vi "sendTwitterCellStats.vi"(8 "error in":errorcluster, 9 "Prev Phase":string, 10 "Prev Exp":T1(ring)=enum."Current Pulse", 11 "cell stats":T2 {"STD" format="%010.2f"; "Variance" format="%010.2f"; "Rt (MOhms)" format="%010.2f"; "tau (ms)" format="%08.2g"; "Cm (pF)" format="%08.2f"; "Ra (MOhms)" format="%010.2f"; "Rm (MOhms)" format="%010.2f"; "Ihold (pA)" format="%010.2f"}) -> (0 "error out":errorcluster, 3 "check Time":timestamp)   [LabVIEW 2019]
uses:
  <vilib>/LVH/i3 Twitter/Controls/Twitter Handle.ctl
  <vilib>/LVH/i3 OAuth/Controls/OAuth Handle.ctl
  <vilib>/LVH/i3 OAuth/Controls/Signature Method.ctl
  <vilib>/LVH/i3 OAuth/Controls/Credentials.ctl
  wc_protocol_v1.003 Folder/whole_cell_protocol/Controls/cell_stats-v02.ctl
  <vilib>/LVH/i3 Twitter/SubVIs/Twitter Open - Embedded.vi
  <vilib>/LVH/i3 Twitter/Tweets/Post Tweet.vi
  <vilib>/LVH/i3 Twitter/i3-twitter.lvlib
  <vilib>/LVH/i3 OAuth/i3-oauth.lvlib
panel:
  out "tweet sent":string
  out "Twitter Handle Out":T3={"OAuth Credentials"={"Signature Method"=enum."HMAC-SHA1", "Version"="1.0", "Client"={"Token"="", "Secret"=""}, "Access"={"Token"="", "Secret"=""}}, "since ID"="", "max ID"="", "Screen Name"=""}
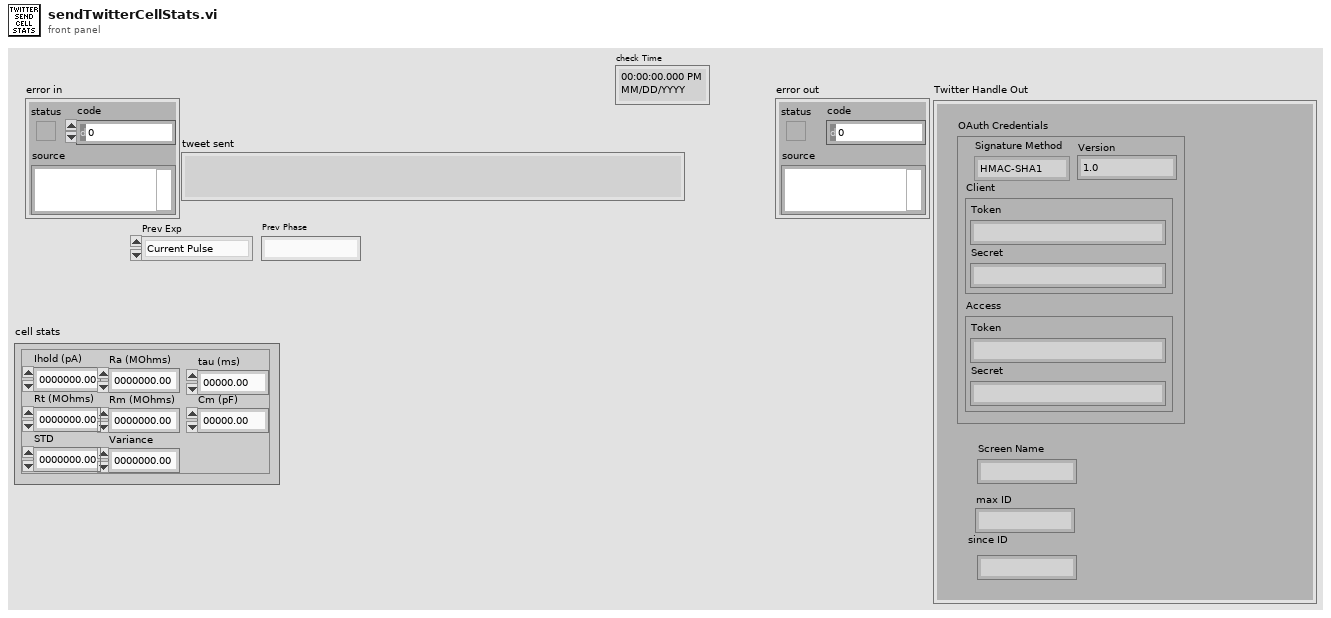
[diagram p1: front panel]
types:
  T1 = enum32{"Single Jump", "Solution Change", "Voltage Step", "Voltage Ramp", "Voltage Pulse", "Jump Train", "Paired Pulse", "Single Manip Jump", "Gap Free", "Multi M. Jump", "Current Pulse", "Current Ramp", "Gap Free Iclamp"}
  T2 = typedef "cell_stats-v02.ctl" = cluster{"Ihold (pA)":dbl, "Rm (MOhms)":dbl, "Ra (MOhms)":dbl, "Cm (pF)":dbl, "tau (ms)":dbl, "Rt (MOhms)":dbl, "Variance":dbl, "STD":dbl}
  T3 = typedef "i3-twitter.lvlib/Twitter Handle.ctl" = cluster{"OAuth Credentials":T4, "since ID":string, "max ID":string, "Screen Name":string}
  T4 = typedef "i3-oauth.lvlib/OAuth Handle.ctl" = cluster{"Signature Method":T5, "Version":string, "Client":T6, "Access":T6}
  T5 = typedef "i3-oauth.lvlib/Signature Method.ctl" = enum16{"HMAC-MD5", "HMAC-SHA1", "HMAC-SHA224", "HMAC-SHA256", "HMAC-SHA384", "HMAC-SHA512"}
  T6 = typedef "i3-oauth.lvlib/Credentials.ctl" = cluster{"Token":string, "Secret":string}
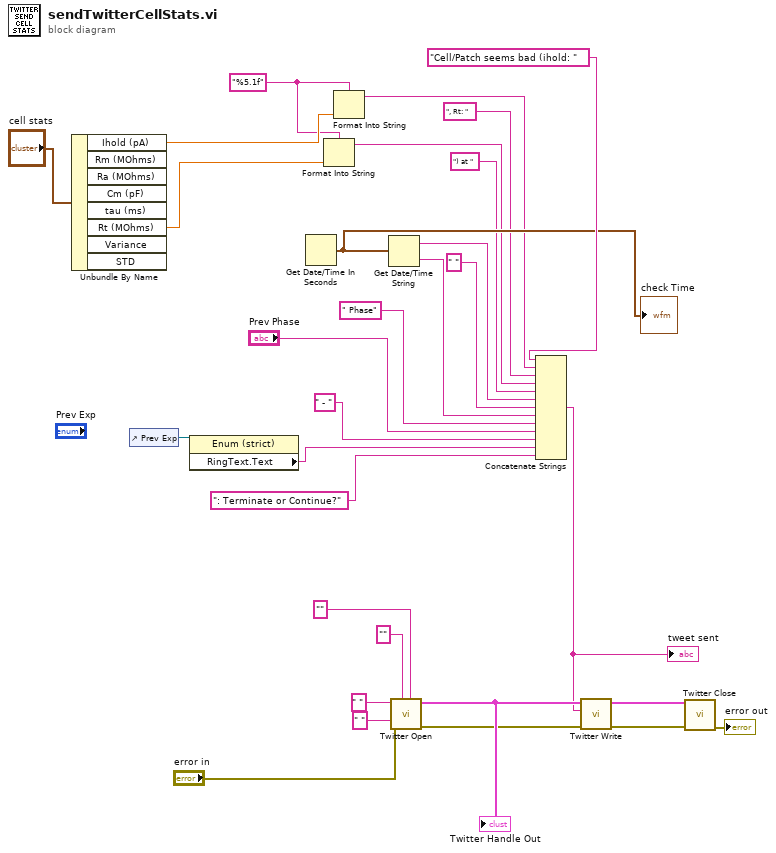
[diagram p0: block diagram]
diagram:
  w1 = "%5.1f" ("format string")
  n1 = Unbundle By Name("cell stats") -> ("Ihold (pA)"=w13:dbl, "Rt (MOhms)"=w11:dbl)  [unwired: 6 out]
  n2 = control-ref of="Prev Exp"() -> (w4:refnum<vi>)
  n3 = property class="Enum (strict)"(reference=w4) -> ("RingText.Text"=w3:string)  [unwired: 1 in, 2 out]
  n4 = Get Date/Time In Seconds() -> (seconds since 1Jan1904=w18:timestamp)
  "check Time" <- w18
  n5 = Format Into String(format string=w1, w11) -> (resulting string=w10:string)  [unwired: 2 in, 1 out]
  n6 = Format Into String(format string=w1, w13) -> (resulting string=w12:string)  [unwired: 2 in, 1 out]
  n7 = Get Date/Time String(seconds (now)=w18) -> (date string=w17:string, time string=w16:string)  [unwired: 2 in]
  n8 = call-poly <vilib>:"Twitter Open.vi"("Access Secret"="", "Access Token"="", "error in"="error in", "Consumer Secret"=" ", "Consumer Key"=" ") -> ("error out"=w25:errorcluster, "Twitter Handle Out"=w26:T3)  [unwired: 5 in]
  "Twitter Handle Out" <- w26
  n9 = Concatenate Strings("Cell/Patch seems bad (ihold: " ("Tweet"), w12, ", Rt: " ("Tweet"), w10, ") at " ("string"), w17, " " ("string"), w16, " Phase" ("string"), "Prev Phase", " - " ("string"), w3, ": Terminate or Continue?" ("string")) -> (w20:string)
  "tweet sent" <- w20
  n10 = call-poly <vilib>:"Twitter Write.vi"("error in (no error)"=w25, "Tweet"=w20, "Twitter Handle In"=w26) -> ("error out"=w23:errorcluster, "Twitter Handle Out"=w24:T3)  [unwired: 7 in]
  n11 = call <vilib>:"Twitter Close.vi"("error in"=w23, "Twitter Handle In"=w24) -> ("error out"=→"error out":errorcluster)  [unwired: 9 in]
